vi "Offset Widget Offset Values.vi"(7 "Force Offset Tag":string, 8 "Coordinate Space":bool caption="Coord", 9 "Rigid Connection In":bool, 10 "Number of\nLBCBs":T1, 11 "Offset Type":T2) -> (3 "Offsets":dbl[][](array[numeric]))   [LabVIEW 2009]
uses:
  Offset Types.ctl
  Data Access Objects/Application/Number Of LBCBs.ctl
  Global Data/Transactions/Dataset Transaction Id.ctl
  Global Data/Transactions/Dataset Source.ctl
  Global Data/Transactions/Dataset Type.ctl
  Apps/Yes No Button.ctl
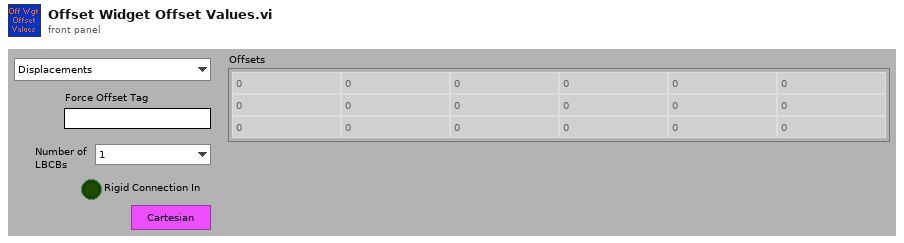
[diagram p1: front panel]
types:
  T1 = typedef "Number Of LBCBs.ctl" = enum16{"1", "2"}
  T2 = typedef "Offset Types.ctl" = enum16{"Displacements", "Forces", "External Sensors"}
  T3 = typedef "Dataset Transaction Id.ctl" = cluster{"Dataset Source":T4, "Dataset Type":T5, "Hold":T6, "Volts":T6, "Tag":string}
  T4 = typedef "Dataset Source.ctl" = enum16{"LBCB 1", "LBCB 2", "Combined", "External Sensors"}
  T5 = typedef "Dataset Type.ctl" = enum16{"LVDT", "Load Cell", "Actuator Command", "Servo Error", "Displacement Command", "Displacement", "Force"}
  T6 = typedef "Yes No Button.ctl" = bool
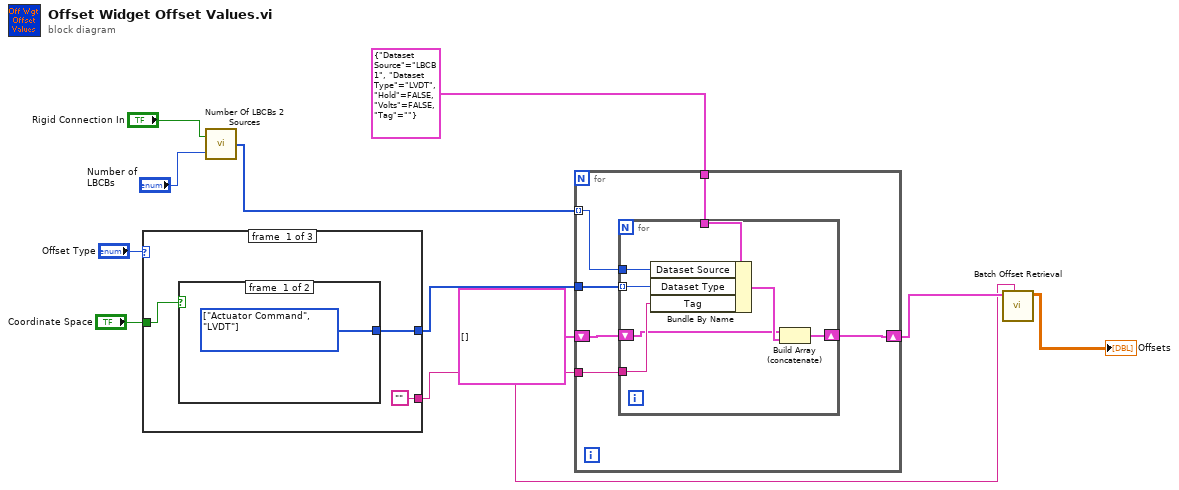
[diagram p0: block diagram]
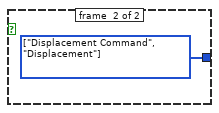
[diagram p2: hidden frame]
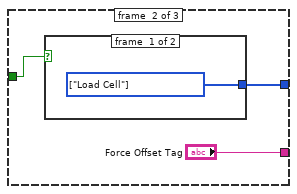
[diagram p3: hidden frame]
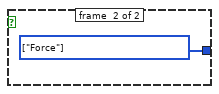
[diagram p4: hidden frame]
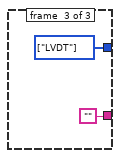
[diagram p5: hidden frame]
diagram:
  n1 = case shown="\"Displacements\"" "Offset Type" {
    tunnel: "Coordinate Space" -> [w14 w19 _]
    tunnel: [w13 w18 w23] -> w5
    tunnel: ["" "Force Offset Tag" ""] -> w2
    frame #0 {
      n2 = case shown="False" w14 {
        tunnel: [w15 w16] -> w13
        frame #0 {
          w15 = T5[] [enum."Actuator Command", enum."LVDT"] items=["LVDT", "Load Cell", "Actuator Command", "Servo Error", "Displacement Command", "Displacement", "Force"]
        }
        frame #1 {
          w16 = T5[] [enum."Displacement Command", enum."Displacement"] items=["LVDT", "Load Cell", "Actuator Command", "Servo Error", "Displacement Command", "Displacement", "Force"]
        }
      }
    }
    frame #1 {
      n3 = case shown="True" w19 {
        tunnel: [w20 w21] -> w18
        frame #0 {
          w20 = T5[] [enum."Load Cell"] items=["LVDT", "Load Cell", "Actuator Command", "Servo Error", "Displacement Command", "Displacement", "Force"]
        }
        frame #1 {
          w21 = T5[] [enum."Force"] items=["LVDT", "Load Cell", "Actuator Command", "Servo Error", "Displacement Command", "Displacement", "Force"]
        }
      }
    }
    frame #2 {
      w23 = T5[] [enum."LVDT"] items=["LVDT", "Load Cell", "Actuator Command", "Servo Error", "Displacement Command", "Displacement", "Force"]
    }
  }
  n4 = call "Number Of LBCBs 2 Sources.vi"("Number of LBCBs"="Number of\nLBCBs", "Combined LBCBs"="Rigid Connection In") -> ("Sources"=w9:T4[])
  n5 = for {
    tunnel: w9 -> [w27] mode=indexing
    tunnel: T3 {"Dataset Source"=enum."LBCB 1", "Dataset Type"=enum."LVDT", "Hold"=FALSE, "Volts"=FALSE, "Tag"=""} ("Dataset Trans Id") -> [w29]
    tunnel: w2 -> [w28]
    tunnel: w5 -> [w26]
    shift-right: [w25] -> w4
    shift-left: T3[] [] -> [w24]
    n6 = for {
      tunnel: w29 -> [w36]
      tunnel: w28 -> [w35]
      tunnel: w27 -> [w34]
      tunnel: w26 -> [w33] mode=indexing
      shift-right: [w31] -> w25
      shift-left: w24 -> [w30]
      n7 = Bundle By Name(cluster=w36, "Dataset Source"=w34, "Dataset Type"=w33, "Tag"=w35) -> (w32:T3)
      n8 = Build Array (concatenate)(w30, w32) -> (w31:T3[])
    }
  }
  n9 = call "Batch Offset Retrieval.vi"("Tag"=w2, "Transactions"=w4) -> ("Data"=→"Offsets":dbl[][])  [unwired: 8 in, 1 out]
